vi "ni579x Repeat Host Driven Synchronization.vi"(0 "Register Buses":T1[](array[typedef]), 7 "synchronization data in valid":bool, 9 "synchronization data in":u16[](array[numeric]), 11 "error in":errorcluster, 12 "sync.cptr.period":u16=13) -> (4 "Register Buses (out)":T1[](array[typedef]), 10 "synchronization data out":u16[](array[numeric]), 15 "error out":errorcluster)   [LabVIEW 2015, in "ni579x Synchronization v2 Host.lvlib"]
doc: "Use this flavor of synchronization in conjunction with \"ni579x Host Align\" on the FPGA. Please refer to the FPGA VIs for documentation. After this VI finishes, the FPGAs will be synchronized. Use this version of synchronization to return to a known synchronization state from a previous run. It is possible for the FPGAs to <B>not be synchronized</B> if the <B>synchronization data in</B> is incorrect. Synchronization data is also only valid for a given system configuration. If FlexRIO FPGA modules, FlexRIO adapter modules, chassis, or slot locations change then synchronization data may not be valid.\n\n<B>Input Parameters</B>\n\n<B>Register Buses</B> specifies the Register Buses to which the Synchronization library is connected in the FPGA VIs.\n\n<B>sync.cptr.period</B> is the period (in clocks) of the Common Periodic Time Reference (CPTR). The CPTR period controls the rate at which synchronized signals are realized. This parameter is optional, and defaults to 13.\n\nWhen using 'ni579x FPGA Align', the CPTR period must be the same as the reference clock period. The 'sync.cptr.period' must be set to the ratio of the Single Cycle Timed Loop (SCTL) rate (that the Alignment VI is in) to the 'sync.meas.Reference Clock' rate. For example, the CPTR period must be 13 if using the PXI_Clk10 for the reference clock, and the IO Module\\Sample Clock for the SCTL clock (130 MHz / 10 MHz).\n\nWhen using 'ni579x Host Align', this value is configurable. The maximum value is 63. The minimum value for the 'sync.cptr.period' must be big enough to ensure transmission across the 'sync.cptr.FPGA I/O' line. Refer to the specifications for the FPGA I/O line chosen. For example, if the FPGA I/O line has a maximum propagation delay of 50ns, then the minimum value would be 7 (the period of the 130 MHz IO Module\\Sample Clock is ~7.692ns, so it would require 7 clocks to exceed 50ns). It is not recommended to change the CPTR period on-the-fly. Alignment must be re-run if the CPTR period is changed.\n\n<B>synchronization data in valid</B> is a flag to use the values from a previous synchronization run ('synchronization data in') to return the FPGAs to that synchronization state.\n\n<B>synchronization data in</B> is the synchronization data from a previous synchronization run that can be used to return the FPGAs to that synchronization state.\n\n<B>error in</B> describes error conditions that occur before this node runs. This input provides standard 'error in' functionality.\n\n<B>Output Parameters</B>\n\n<B>Register Buses (out)</B> passes the Register Buses to the next VI.\n\n<B>synchronization data out</B> is the data from this synchronization run. This data can be used to return the FPGAs to this synchronization state. This data is only valid if the FPGAs were successfully synchronized (no output error).\n\n<B>error out</B> contains error information. This output provides standard 'error out' functionality."
uses:
  <instrlib>/ni579x/Synchronization/v2/Host/ni579x Synchronization v2 Host.lvlib
  <instrlib>/_niInstr/Register Bus/v0/Host/Public/Register Bus Session.ctl
  <instrlib>/_niInstr/Register Bus/v0/Host/Private/Session Data.ctl
  <instrlib>/_niInstr/Register Bus/v0/Host/niInstr Register Bus v0 Host.lvlib
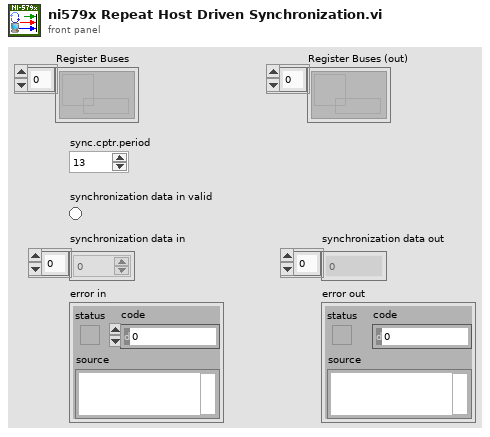
[diagram p1: front panel]
types:
  T1 = typedef "niInstr Register Bus v0 Host.lvlib/Register Bus Session.ctl" = refnum<queue>
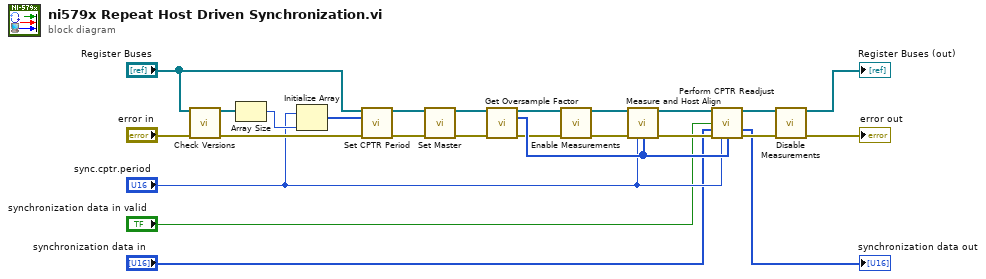
[diagram p0: block diagram]
diagram:
  n1 = call <instrlib>:"Check Versions.vi"("Register Buses"="Register Buses", "error in"="error in") -> ("Register Buses (out)"=w9:T1[], "error out"=w11:errorcluster)  [unwired: 12 in]
  n2 = Array Size(array=w9) -> (size(s)=w16:i32)
  n3 = Initialize Array("sync.cptr.period", w16) -> (w17:u16[])
  n4 = call <instrlib>:"Set CPTR Period.vi"("Register Buses"="Register Buses", "sync.cptr.period"=w17, "error in"=w11) -> ("Register Buses (out)"=w18:T1[], "error out"=w19:errorcluster)  [unwired: 11 in]
  n5 = call <instrlib>:"Set Master.vi"("Register Buses"=w18, "error in"=w19) -> ("Register Buses (out)"=w8:T1[], "error out"=w15:errorcluster)  [unwired: 12 in]
  n6 = call <instrlib>:"Get Oversample Factor.vi"("Register Buses"=w8, "error in"=w15) -> ("Register Buses (out)"=w13:T1[], "sync.meas.oversample factor"=w25:u16[], "error out"=w14:errorcluster)  [unwired: 11 in]
  n7 = call <instrlib>:"Enable Measurements.vi"("Register Buses"=w13, "error in"=w14) -> ("Register Buses (out)"=w20:T1[], "error out"=w22:errorcluster)  [unwired: 12 in]
  n8 = call <instrlib>:"Measure and Host Align.vi"("Register Buses"=w20, "error in"=w22, "sync.cptr.period"="sync.cptr.period", "sync.meas.oversample factor"=w25) -> ("Register Buses (out)"=w6:T1[], "error out"=w24:errorcluster)  [unwired: 10 in]
  n9 = call <instrlib>:"Perform CPTR Readjust.vi"("Register Buses"=w6, "synchronization data in valid"="synchronization data in valid", "synchronization data in"="synchronization data in", "error in"=w24, "sync.cptr.period"="sync.cptr.period", "sync.meas.oversample factor"=w25) -> ("Register Buses (out)"=w5:T1[], "synchronization data"=→"synchronization data out":u16[], "error out"=w7:errorcluster)  [unwired: 7 in]
  n10 = call <instrlib>:"Disable Measurements.vi"("Register Buses"=w5, "error in"=w7) -> ("Register Buses (out)"=→"Register Buses (out)":T1[], "error out"=→"error out":errorcluster)  [unwired: 12 in]
